vi "SigMath Class - Close ALL Window.vi"(5 "error in (no error)":errorcluster) -> (19 "error out":errorcluster)   [LabVIEW 2022 SP3, in "SigMath.lvclass"]
uses:
  SigMath.lvclass
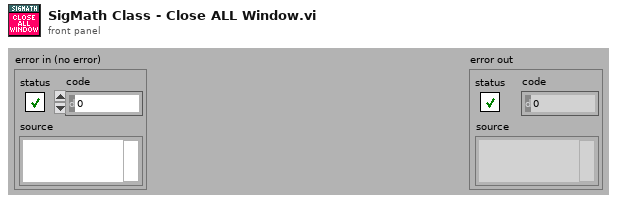
[diagram p1: front panel]
types:
  T1 = typedef "SigMath.lvclass/ClassAttributes.ctl" = cluster{"Window List":refnum<vi>[]}
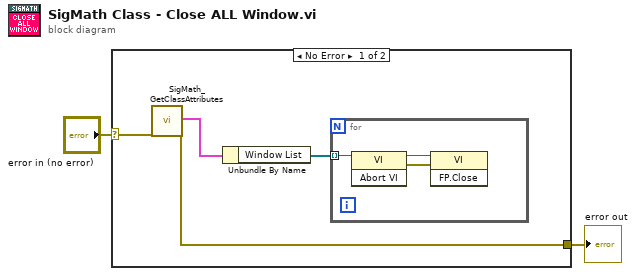
[diagram p0: block diagram]
diagram:
  n1 = case shown="No Error" "error in (no error)" {
    selector: "error in (no error)" -> [w6 w10]
    tunnel: [w5 w10] -> w1
    frame No Error {
      n2 = call "SigMath_GetClassAttributes.vi"("error in (no error)"=w6) -> ("class attributes"=w4:T1, "error out"=w5:errorcluster)  [unwired: 15 in, 2 out]
      n3 = Unbundle By Name(w4) -> ("Window List"=w3:refnum<vi>[])
      n4 = for {
        tunnel: w3 -> [w9] mode=indexing
        n5 = invoke class="VI" method="Abort VI"(reference=w9) -> (reference out=w8:refnum<vi>, error out=w7:errorcluster)  [unwired: 2 in, 1 out]
        n6 = invoke class="VI" method="FP.Close"(reference=w8, error in=w7) -> ()  [unwired: 1 in, 3 out]
      }
    }
    frame Error {
    }
  }
  "error out" <- w1
